vi "Write AttrName.vi"(10 "Attribute Name":string, 11 "Attribute in":refnum<class "Attribute.lvclass">) -> (3 "Attribute out":refnum<class "Attribute.lvclass">)   [LabVIEW 2013, in "SMOAttributes.lvlib" / "Attribute.lvclass"]
uses:
  Attribute.lvclass
  Attribute.lvclass/Attribute.ctl
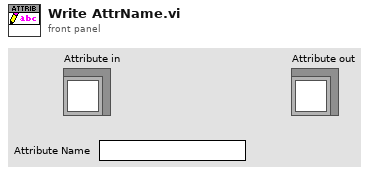
[diagram p1: front panel]
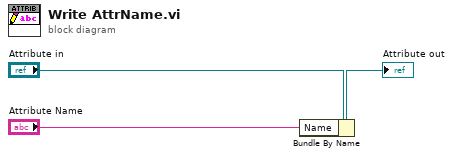
[diagram p0: block diagram]
diagram:
  n1 = Bundle By Name(cluster="Attribute in", "Name"="Attribute Name") -> (→"Attribute out":refnum<class "Attribute.lvclass">)
